vi "slowinit.vi"(8 "UTC format":bool=TRUE, 9 "XOFF Character":u8=19 format="%.0x", 10 "XON Character":u8=17 format="%.0x", 11 "VISA resource name":refnum<visa-resource-name>="COM5") -> (0 "error IO":errorcluster, 3 "VISA resource name out":refnum<visa-resource-name>, 6 "Number of Slow Parameters":i32, 7 "Slow Cluster":T1={"Number of Slow Parameters"=0, "UTC format?"=TRUE, "Sensor Upper bounds"=[85, 1000000, 8000, 8000, 8000, 14000, 99, 33000], "Sensor Lower bounds"=[-40, 0, -8000, -8000, -8000, -14000, 0, -33000], "datanames"=[], "Descriptions"=[]})   [LabVIEW 2012]
uses:
  <vilib>/Instr/_visa.llb/VISA Configure Serial Port (Instr).vi
panel:
  out "Stopped":bool
  out "array of datanames":string[](array[string])
  out "array of datanames 2":string[](array[string])
  out "Arduino needs to be reinitialized":bool
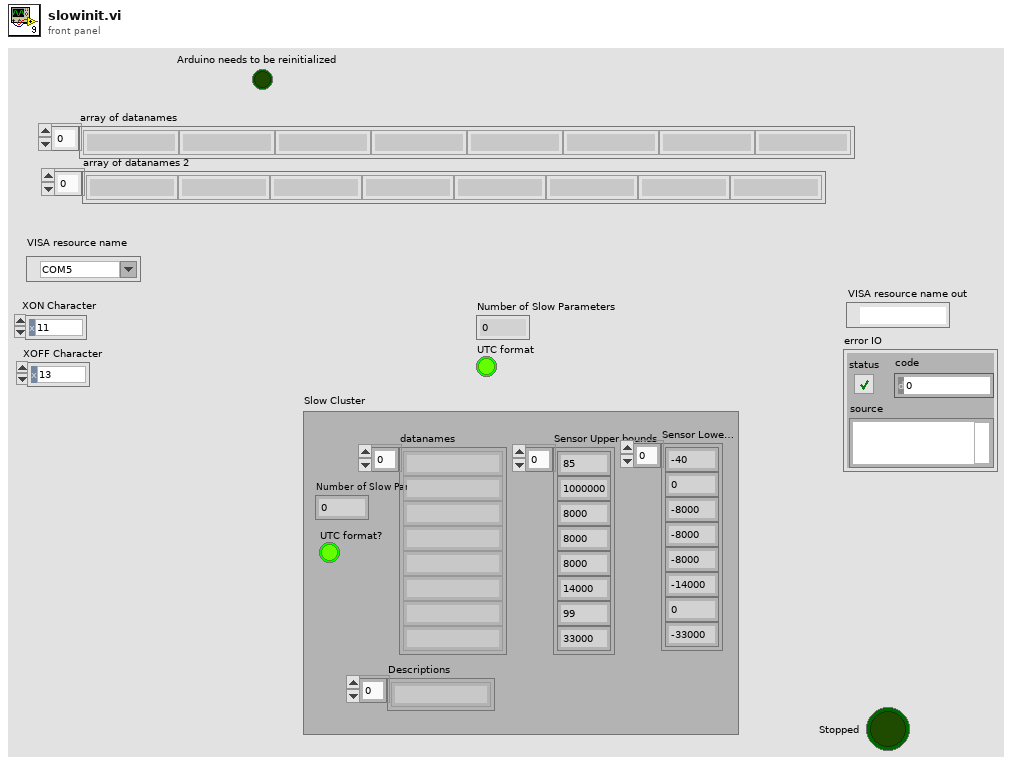
[diagram p1: front panel]
types:
  T1 = cluster{"Number of Slow Parameters":i32, "UTC format?":bool, "Sensor Upper bounds":i32[], "Sensor Lower bounds":i32[], "datanames":string[], "Descriptions":string[]}
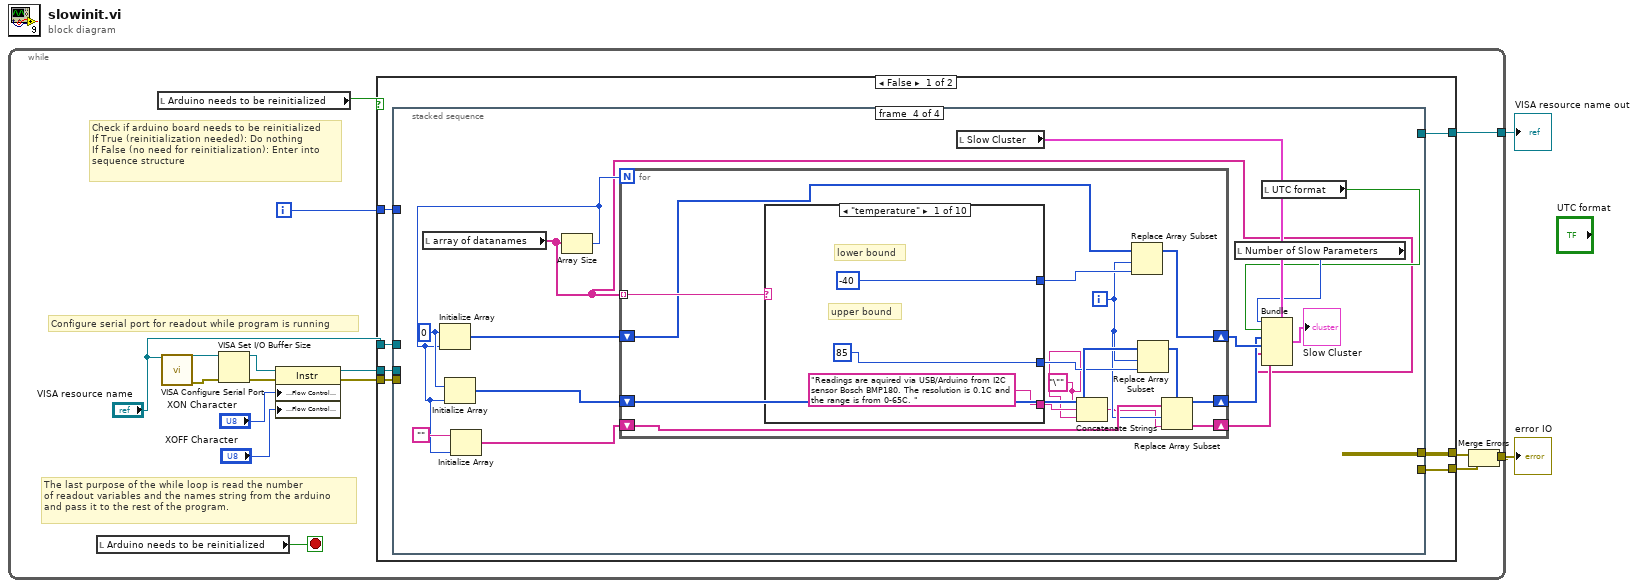
[diagram p0: block diagram]
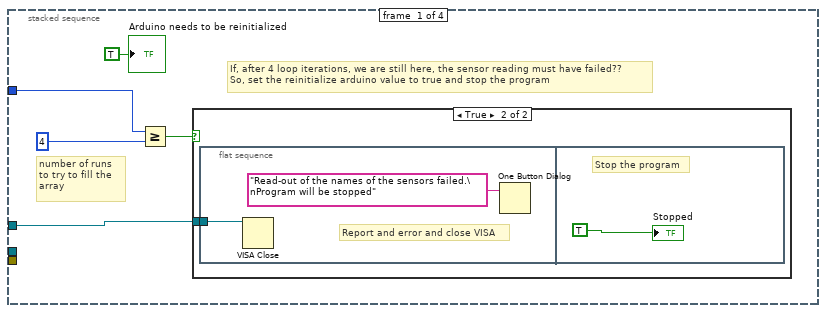
[diagram p2: hidden frame]
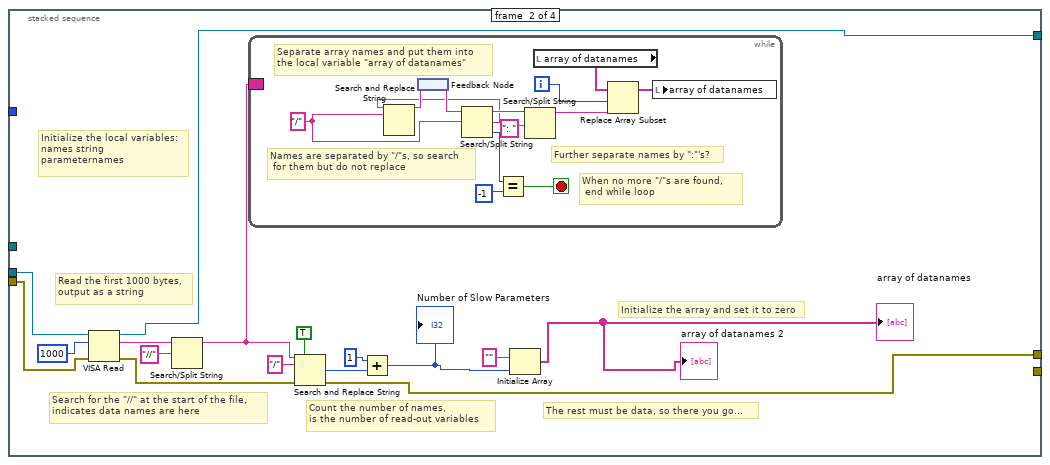
[diagram p4: hidden frame]
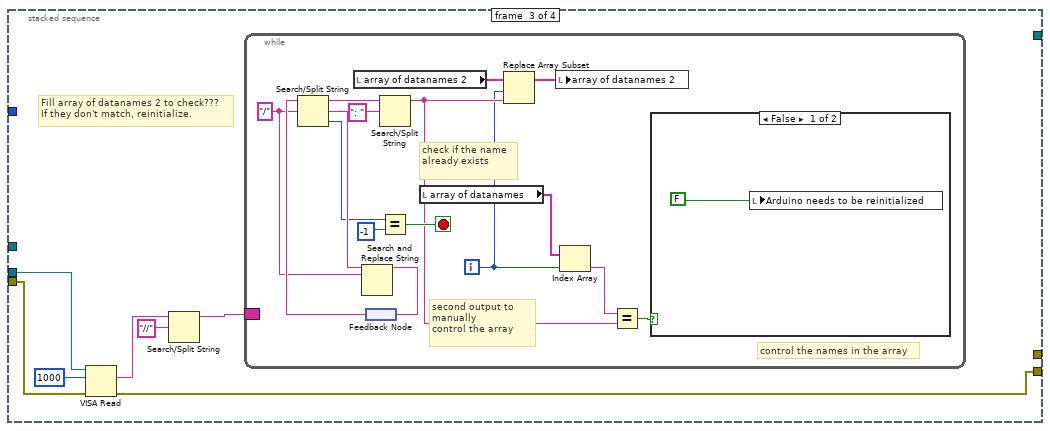
[diagram p5: hidden frame]
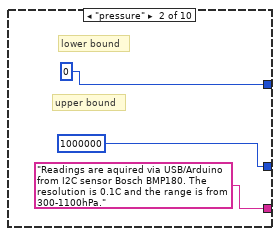
[diagram p7: hidden frame]
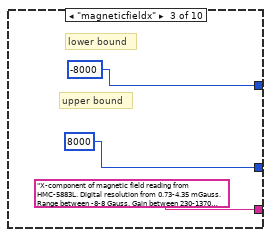
[diagram p8: hidden frame]
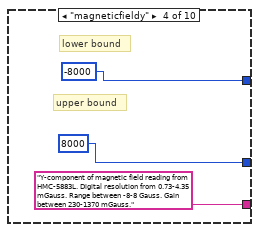
[diagram p9: hidden frame]
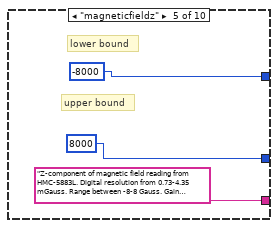
[diagram p10: hidden frame]
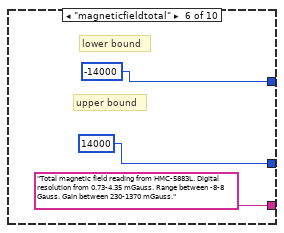
[diagram p11: hidden frame]
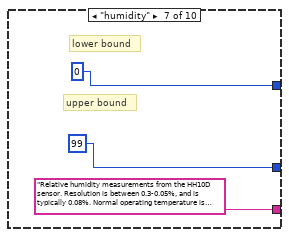
[diagram p12: hidden frame]
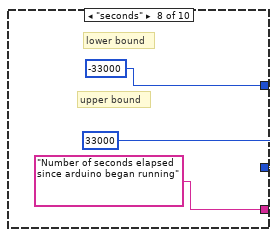
[diagram p13: hidden frame]
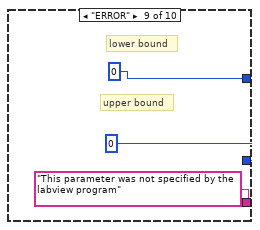
[diagram p14: hidden frame]
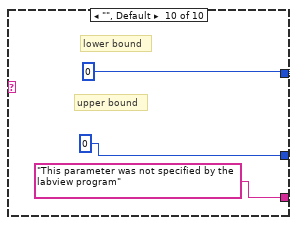
[diagram p15: hidden frame]
diagram:
  n1 = while {
    tunnel: [w12] -> w2
    tunnel: [w11] -> w1
    i -> [w9]
    stop <- w7 stop-if-true
    # "The last purpose of the while loop is read the number \nof readout variables and the names string from the arduino\nand pass it to the rest of the program."
    # "Check if arduino board needs to be reinitialized\nIf True (reinitialization needed): Do nothing\nIf False (no need for reinitialization): Enter into \nsequence structure"
    # "Configure serial port for readout while program is running"
    n2 = local read "Arduino needs to be reinitialized"() -> (w7:bool)
    n3 = local read "Arduino needs to be reinitialized"() -> (w6:bool)
    n4 = call-poly "VISA Configure Serial Port"("VISA resource name"="VISA resource name") -> ("VISA resource name out"=w14:refnum<visa-resource-name>, "error out"=w13:errorcluster)  [unwired: 9 in, 4 out]
    n5 = VISA Set I/O Buffer Size(VISA resource name=w14, error in (no error)=w13) -> (VISA resource name out=w18:refnum<visa-resource-name>, error out=w17:errorcluster)  [unwired: 2 in]
    n6 = property class="Instr"(reference=w18, error in=w17, "Serial Settings:Flow Control XON Character"="XON Character", "Serial Settings:Flow Control XOFF Character"="XOFF Character") -> (reference out=w10:refnum<visa-resource-name>, error out=w5:errorcluster)
    n7 = case shown="False" w6 {
      tunnel: [w25 w145] -> w12
      tunnel: w10 -> [w24 w145]
      tunnel: w9 -> [w23 _]
      tunnel: "VISA resource name" -> [w22 _]
      tunnel: w5 -> [w21 _]
      tunnel: [w20 _] -> w4
      tunnel: [w19 _] -> w3
      frame False {
        n8 = stacked-sequence {
          tunnel: [_ w47 _ _] -> w25
          tunnel: w24 -> [_ w50 w67 _]
          tunnel: w23 -> [w30 _ _ _]
          tunnel: w22 -> [w27 _ _ _]
          tunnel: w21 -> [_ w48 w65 _]
          tunnel: [_ w37 _ _] -> w20
          tunnel: [_ _ w64 _] -> w19
          frame #0 {
            # "If, after 4 loop iterations, we are still here, the sensor reading must have failed??  \nSo, set the reinitialize arduino value to true and stop the program"
            # "number of runs to try to fill the array"
            n9 = Greater Or Equal?(x=w30, y=4) -> (x >= y?=w28:bool)
            n10 = case shown="True" w28 {
              tunnel: w27 -> [_ w31]
              frame False {
              }
              frame True {
                n11 = flat-sequence {
                  tunnel: w31 -> [w32]
                  frame #0 {
                    # "Report and error and close VISA"
                    n12 = VISA Close(VISA resource name=w32) -> ()  [unwired: 1 in, 1 out]
                    n13 = One Button Dialog(message="Read-out of the names of the sensors failed.\nProgram will be stopped") -> ()  [unwired: 1 in, 1 out]
                  }
                  frame #1 {
                    # "Stop the program"
                    "Stopped" <- TRUE ("stop? (T)")
                  }
                }
              }
            }
            "Arduino needs to be reinitialized" <- TRUE ("Arduino needs to be reinitialized")
          }
          frame #1 {
            # "The rest must be data, so there you go..."
            # "Count the number of names, \nis the number of read-out variables"
            # "Search for the \"//\" at the start of the file, \nindicates data names are here"
            # "Initialize the local variables: \nnames string\nparameternames"
            # "Read the first 1000 bytes, \noutput as a string"
            # "Initialize the array and set it to zero"
            n14 = VISA Read(VISA resource name=w50, byte count=u32 1000, error in (no error)=w48) -> (VISA resource name out=w47:refnum<visa-resource-name>, read buffer=w46:string, error out=w38:errorcluster)  [unwired: 1 out]
            n15 = Search/Split String(string=w46, search string/char (-)="//") -> (substring before match=w42:string)  [unwired: 1 in, 2 out]
            n16 = while {
              border: w42 -> [_]
              i -> [w51]
              stop <- w60 stop-if-true
              w56 = "/" ("search string/char (-)")
              # "Further separate names by \":\"'s?"
              # "When no more \"/\"s are found,\n end while loop"
              # "Names are separated by \"/\"s, so search\n for them but do not replace"
              # "Separate array names and put them into \nthe local variable \"array of datanames\""
              n17 = feedback #1() -> (w58:string)
              n18 = Search/Split String(string=w58, search string/char (-)=w56) -> (substring before match=w54:string, match + rest of string=w53:string, offset of match=w55:i32)  [unwired: 1 in]
              n19 = Search and Replace String(input string=w53, search string=w56) -> (result string=w57:string)  [unwired: 6 in, 3 out]
              n20 = feedback-in #1(w57) -> ()
              n21 = Equal?(x=w55, y=-1) -> (x = y?=w60:bool)
              n22 = Search/Split String(string=w54, search string/char (-)=": " ("format string")) -> (substring before match=w52:string)  [unwired: 1 in, 2 out]
              n23 = local read "array of datanames"() -> (w62:string[])
              n24 = Replace Array Subset(array=w62, new element=w52, index=w51) -> (w61:string[])
              n25 = local write "array of datanames"(w61) -> ()
            }
            n26 = Search and Replace String(replace all?=TRUE ("replace all? (F)"), input string=w42, search string="/", error in=w38) -> (number of replacements=w43:i32, error out=w37:errorcluster)  [unwired: 4 in, 2 out]
            n27 = Add(x=1, y=w43) -> (x+y=w36:i32)
            "Number of Slow Parameters" <- w36
            n28 = Initialize Array("", w36) -> (→"array of datanames" →"array of datanames 2":string[])
          }
          frame #2 {
            # "Fill array of datanames 2 to check???\nIf they don't match, reinitialize."
            n29 = VISA Read(VISA resource name=w67, byte count=u32 1000, error in (no error)=w65) -> (read buffer=w70:string, error out=w64:errorcluster)  [unwired: 2 out]
            n30 = Search/Split String(string=w70, search string/char (-)="//") -> (substring before match=w66:string)  [unwired: 1 in, 2 out]
            n31 = while {
              border: w66 -> [_]
              i -> [w71]
              stop <- w82 stop-if-true
              w77 = "/" ("search string/char (-)")
              # "second output to manually\ncontrol the array"
              # "check if the name already exists"
              # "control the names in the array"
              n32 = local read "array of datanames 2"() -> (w84:string[])
              n33 = feedback #2() -> (w80:string)
              n34 = Search/Split String(string=w80, search string/char (-)=w77) -> (substring before match=w85:string, match + rest of string=w79:string, offset of match=w76:i32)  [unwired: 1 in]
              n35 = Search and Replace String(input string=w79, search string=w77) -> (result string=w78:string)  [unwired: 6 in, 3 out]
              n36 = feedback-in #2(w78) -> ()
              n37 = Search/Split String(string=w85, search string/char (-)=": " ("format string")) -> (substring before match=w73:string)  [unwired: 1 in, 2 out]
              n38 = Equal?(x=w76, y=-1) -> (x = y?=w82:bool)
              n39 = local read "array of datanames"() -> (w74:string[])
              n40 = Replace Array Subset(array=w84, new element=w73, index=w71) -> (w83:string[])
              n41 = local write "array of datanames 2"(w83) -> ()
              n42 = Index Array(array=w74, index=w71) -> (element=w75:string)
              n43 = Equal?(x=w75, y=w73) -> (x = y?=w72:bool)
              n44 = case shown="False" w72 {
                frame False {
                  n45 = local write "Arduino needs to be reinitialized"(FALSE ("reinitialize arduino read boolean")) -> ()
                }
                frame True {
                }
              }
            }
          }
          frame #3 {
            w101 = 0 ("element")
            n46 = local read "array of datanames"() -> (w88:string[])
            n47 = Array Size(array=w88) -> (size(s)=w97:i32)
            n48 = Initialize Array(w101, w97) -> (w100:i32[])
            n49 = Initialize Array(w101, w97) -> (w99:i32[])
            n50 = Initialize Array("", w97) -> (w96:string[])
            n51 = for {
              N: w97 -> [_]
              tunnel: w88 -> [w114] mode=indexing
              shift-right: [w108] -> w93
              shift-left: w99 -> [w112]
              shift-right: [w109] -> w94
              shift-left: w100 -> [w113]
              shift-right: [w105] -> w89
              shift-left: w96 -> [w107]
              i -> [w106]
              w103 = "\"" ("string")
              n52 = case shown="\"temperature\"" w114 {
                tunnel: [85 1000000 8000 8000 8000 14000 99 33000 0 0] -> w110
                tunnel: [-40 0 -8000 -8000 -8000 -14000 0 -33000 0 0] -> w111
                tunnel: ["Readings are aquired via USB/Arduino from I2C sensor Bosch BMP180. The resolution is 0.1C and the range is from 0-65C. " "Readings are aquired via USB/Arduino from I2C sensor Bosch BMP180. The resolution is 0.1C and the range is from 300-1100hPa." "X-component of magnetic field reading from HMC-5883L. Digital resolution from 0.73-4.35 mGauss. Range between -8-8 Gauss. Gain between 230-1370 mGauss. " "Y-component of magnetic field reading from HMC-5883L. Digital resolution from 0.73-4.35 mGauss. Range between -8-8 Gauss. Gain between 230-1370 mGauss." "Z-component of magnetic field reading from HMC-5883L. Digital resolution from 0.73-4.35 mGauss. Range between -8-8 Gauss. Gain between 230-1370 mGauss." "Total magnetic field reading from HMC-5883L. Digital resolution from 0.73-4.35 mGauss. Range between -8-8 Gauss. Gain between 230-1370 mGauss." "Relative humidity measurements from the HH10D sensor. Resolution is between 0.3-0.05%, and is typically 0.08%. Normal operating temperature is 0-60C and the drift over time is 1% per year. " "Number of seconds elapsed since arduino began running" ("XML Tag") "This parameter was not specified by the labview program" ("XML Tag") "This parameter was not specified by the labview program" ("XML Tag")] -> w104
                frame "temperature" {
                  # "upper bound"
                  # "lower bound"
                }
                frame "pressure" {
                  # "upper bound"
                  # "lower bound"
                }
                frame "magneticfieldx" {
                  # "upper bound"
                  # "lower bound"
                }
                frame "magneticfieldy" {
                  # "upper bound"
                  # "lower bound"
                }
                frame "magneticfieldz" {
                  # "upper bound"
                  # "lower bound"
                }
                frame "magneticfieldtotal" {
                  # "upper bound"
                  # "lower bound"
                }
                frame "humidity" {
                  # "upper bound"
                  # "lower bound"
                }
                frame "seconds" {
                  # "upper bound"
                  # "lower bound"
                }
                frame "ERROR" {
                  # "upper bound"
                  # "lower bound"
                }
                frame "", Default {
                  # "upper bound"
                  # "lower bound"
                }
              }
              n53 = Concatenate Strings(w103, w104, w103) -> (w102:string)
              n54 = Replace Array Subset(array=w113, new element=w111, index=w106) -> (w109:i32[])
              n55 = Replace Array Subset(array=w112, new element=w110, index=w106) -> (w108:i32[])
              n56 = Replace Array Subset(array=w107, new element=w102, index=w106) -> (w105:string[])
            }
            n57 = local read "Slow Cluster"() -> (w95:T1)
            n58 = local read "Number of Slow Parameters"() -> (w91:i32)
            n59 = local read "UTC format"() -> (w90:bool)
            n60 = Bundle(cluster=w95, "Number of Slow Parameters"=w91, "UTC format?"=w90, "Sensor Upper bounds"=w93, "Sensor Lower bounds"=w94, "datanames"=w88, "Descriptions"=w89) -> (→"Slow Cluster":T1)
          }
        }
      }
      frame True {
      }
    }
    n61 = Merge Errors(w4, w3) -> (w11:errorcluster)
  }
  "VISA resource name out" <- w2
  "error IO" <- w1
